vi "Check_name.vi"(1 "Original file Path":path) -> ()   [LabVIEW 2010]
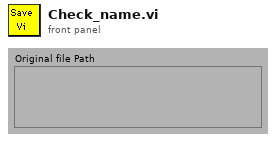
[diagram p1: front panel]
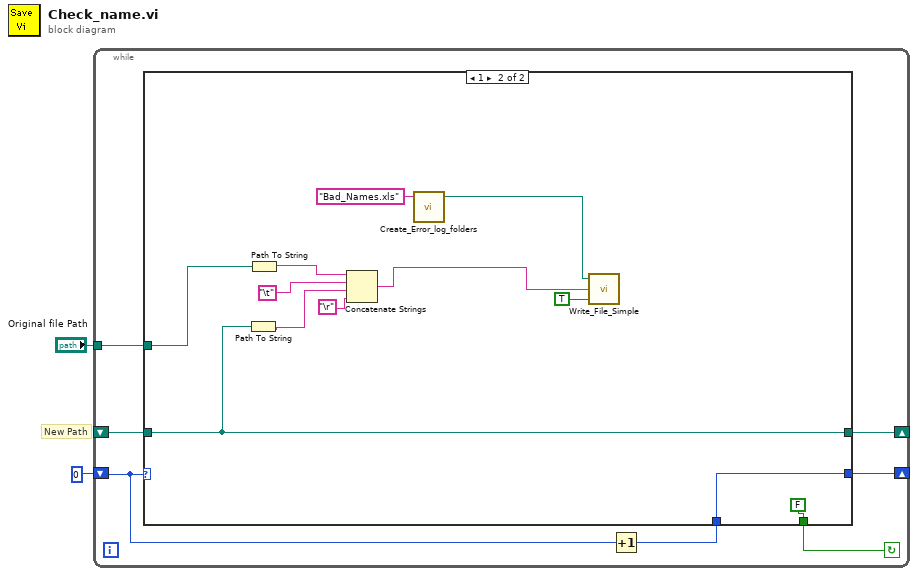
[diagram p0: block diagram]
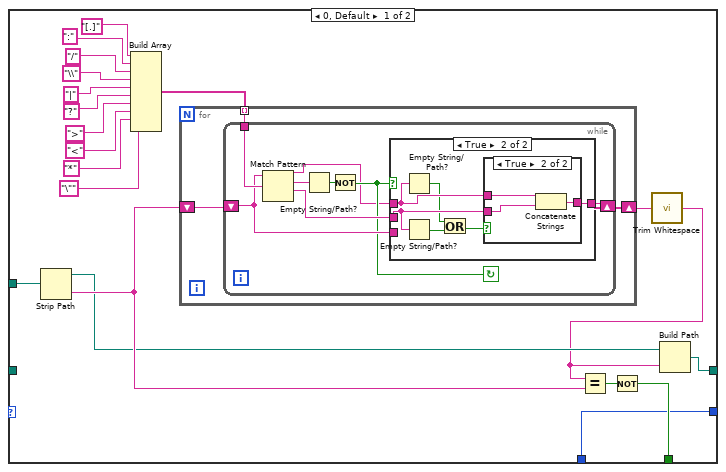
[diagram p2: hidden frame]
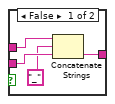
[diagram p4: hidden frame]
diagram:
  # "New Path"
  n1 = while {
    tunnel: "Original file Path" -> [w5]
    shift-left: _ -> [w3]
    shift-right: [w4] -> _
    shift-left: 0 -> [w8]
    shift-right: [w6] -> _
    stop <- w9 continue-if-true
    n2 = Increment(x=w8) -> (x+1=w7:i32)
    n3 = case shown="1" w8 {
      tunnel: [w17 FALSE] -> w9
      tunnel: w7 -> [w16 w66]
      tunnel: [w16 w66] -> w6
      tunnel: w5 -> [w29 w64]
      tunnel: [w19 w63] -> w4
      tunnel: w3 -> [_ w63]
      frame 0, Default {
        n4 = Strip Path(path=w29) -> (stripped path=w20:path, name=w21:string)
        n5 = Build Array("[.]", ":", "/", "\\", "|", "?", ">", "<", "*", "\"") -> (w28:string[])
        n6 = for {
          tunnel: w28 -> [w32] mode=indexing
          shift-right: [w30] -> w15
          shift-left: w21 -> [w31]
          n7 = while {
            shift-left: w31 -> [w36]
            shift-right: [w37] -> w30
            tunnel: w32 -> [w40]
            stop <- w34 continue-if-true
            n8 = Match Pattern(string=w36, regular expression=w40) -> (before substring=w33:string, match substring=w39:string, after substring=w35:string)  [unwired: 2 out]
            n9 = Empty String/Path?(string/path=w39) -> (empty?=w38:bool)
            n10 = Not(x=w38) -> (.not. x?=w34:bool)
            n11 = case shown="True" w34 {
              tunnel: [w41 w42] -> w37
              tunnel: w36 -> [w41 _]
              tunnel: w33 -> [_ w47]
              tunnel: w35 -> [_ w46]
              frame False {
              }
              frame True {
                n12 = Empty String/Path?(string/path=w47) -> (empty?=w44:bool)
                n13 = Empty String/Path?(string/path=w46) -> (empty?=w45:bool)
                n14 = Or(x=w44, y=w45) -> (x .or. y?=w43:bool)
                n15 = case shown="True" w43 {
                  tunnel: w47 -> [w51 w53]
                  tunnel: [w48 w54] -> w42
                  tunnel: w46 -> [w50 w52]
                  frame False {
                    n16 = Concatenate Strings(w51, "_" ("After  Matched string"), w50) -> (w48:string)
                  }
                  frame True {
                    n17 = Concatenate Strings(w53, w52) -> (w54:string)
                  }
                }
              }
            }
          }
        }
        n18 = call <vilib>:"Trim Whitespace.vi"("string"=w15) -> ("trimmed string"=w14:string)  [unwired: 1 in]
        n19 = Equal?(x=w14, y=w21) -> (x = y?=w18:bool)
        n20 = Not(x=w18) -> (.not. x?=w17:bool)
        n21 = Build Path(base path=w20, name or relative path=w14) -> (appended path=w19:path)
      }
      frame 1 {
        n22 = Path To String(path=w63) -> (string=w60:string)
        n23 = Path To String(path=w64) -> (string=w62:string)
        n24 = Concatenate Strings(w62, "\t", w60, "\r") -> (w56:string)
        n25 = call "Create_Error_log_folders.vi"("Log Filename"="Bad_Names.xls") -> ("Local Log File"=w57:path)  [unwired: 2 in, 2 out]
        n26 = call "Write_File_Simple.vi"("append to file? (new file:F)"=TRUE, "character string"=w56, "file path"=w57) -> ()  [unwired: 2 out]
      }
    }
  }
